vi "GetEnterExitLevelofPFLA.vi"(8 "error in (no error)":errorcluster, 10 "DataGroup":T1, 11 "PFLA Source":string) -> (0 "error out":errorcluster, 2 "ExitStartupPFLA%":dbl, 3 "EnterStartupPFLA%":dbl)   [LabVIEW 2017, in "McsaStartupAnalysis.lvlib"]
uses:
  <vilib>/addons/InsightCM/Devices/Shared/Mcsa/McsaStartupAnalysis/McsaStartupAnalysis.lvlib
  <vilib>/addons/InsightCM/MessageBus/Base/controls/R2_DataGroup.ctl
  <vilib>/addons/InsightCM/MessageBus/Base/controls/OperatingState.ctl
  <vilib>/addons/InsightCM/MessageBus/Base/controls/KeyValuePair.ctl
  <vilib>/addons/InsightCM/MessageBus/Base/controls/Trigger.ctl
  <vilib>/addons/InsightCM/MessageBus/Base/controls/Condition.ctl
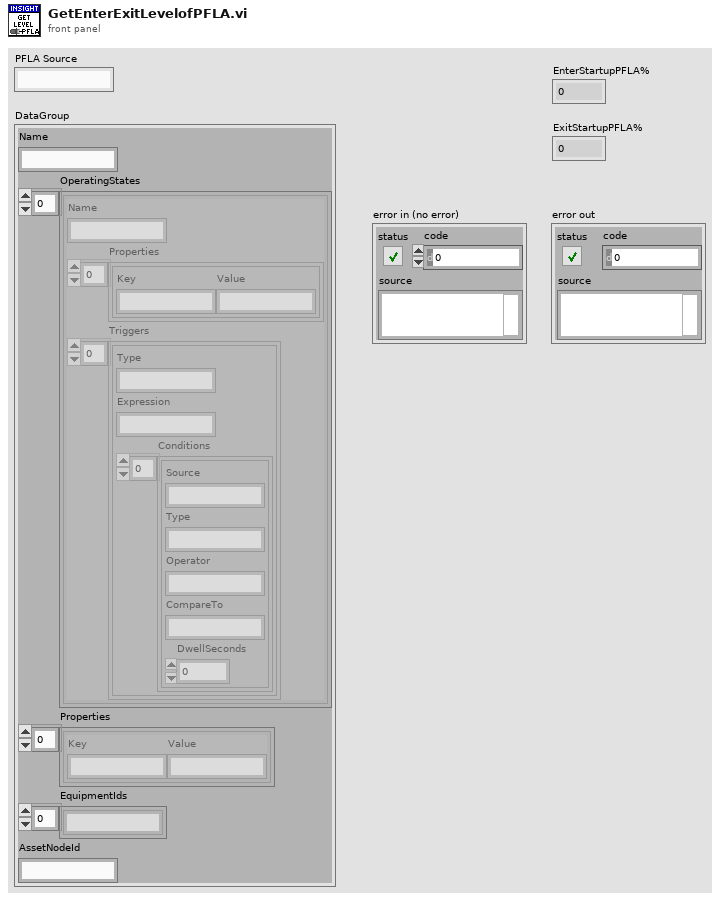
[diagram p1: front panel]
types:
  T1 = typedef "R2_DataGroup.ctl" = cluster{"Name":string, "OperatingStates":T2[], "Properties":T3[], "EquipmentIds":string[], "AssetNodeId":string}
  T2 = typedef "OperatingState.ctl" = cluster{"Name":string, "Properties":T3[], "Triggers":T4[]}
  T3 = typedef "KeyValuePair.ctl" = cluster{"Key":string, "Value":string}
  T4 = typedef "Trigger.ctl" = cluster{"Type":string, "Expression":string, "Conditions":T5[]}
  T5 = typedef "Condition.ctl" = cluster{"Source":string, "Type":string, "Operator":string, "CompareTo":string, "DwellSeconds":dbl}
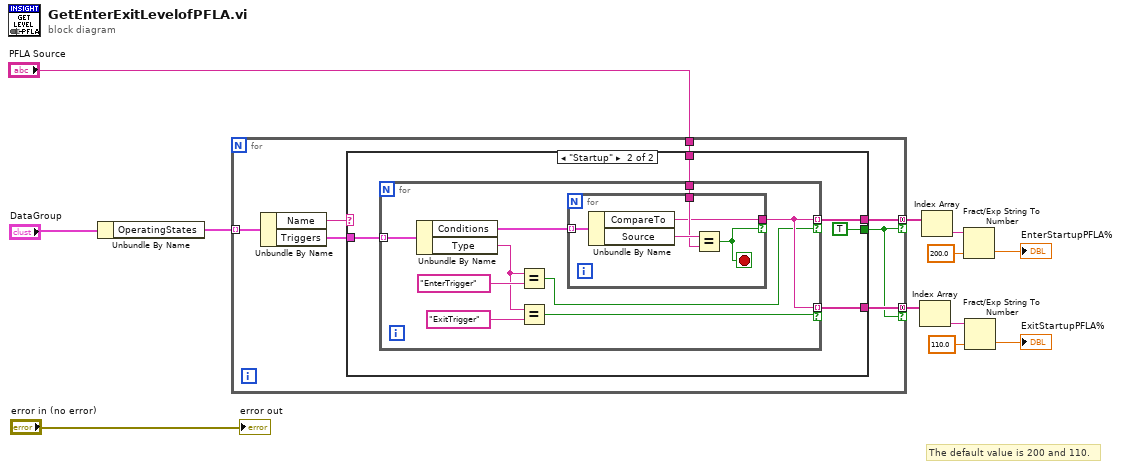
[diagram p0: block diagram]
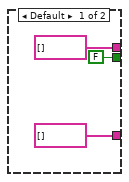
[diagram p2: hidden frame]
diagram:
  # "The default value is 200 and 110."
  n1 = Unbundle By Name("DataGroup") -> ("OperatingStates"=w3:T2[])
  n2 = for {
    tunnel: w3 -> [w19] mode=indexing
    tunnel: "PFLA Source" -> [w17]
    tunnel: [w15] -> w7 mode=concatenating if=w13
    tunnel: [w14] -> w8 mode=concatenating if=w13
    n3 = Unbundle By Name(w19) -> ("Name"=w16:string, "Triggers"=w18:T4[])
    n4 = case shown="\"Startup\"" w16 {
      tunnel: w18 -> [_ w27]
      tunnel: w17 -> [_ w26]
      tunnel: [string[] [] w25] -> w15
      tunnel: [string[] [] w24] -> w14
      tunnel: [FALSE ("x = y?") TRUE ("x = y?")] -> w13
      frame Default {
      }
      frame "Startup" {
        n5 = for {
          tunnel: w27 -> [w36] mode=indexing
          tunnel: w26 -> [w33]
          tunnel: [w30] -> w25 mode=indexing if=w29
          tunnel: [w30] -> w24 mode=indexing if=w28
          n6 = Unbundle By Name(w36) -> ("Conditions"=w34:T5[], "Type"=w31:string)
          n7 = Equal?(x=w31, y="EnterTrigger" ("Type")) -> (x = y?=w29:bool)
          n8 = Equal?(x=w31, y="ExitTrigger" ("Type")) -> (x = y?=w28:bool)
          n9 = for {
            tunnel: w34 -> [w41] mode=indexing
            tunnel: w33 -> [w39]
            tunnel: [w38] -> w30 if=w37
            stop <- w37 stop-if-true
            n10 = Unbundle By Name(w41) -> ("CompareTo"=w38:string, "Source"=w40:string)
            n11 = Equal?(x=w40, y=w39) -> (x = y?=w37:bool)
          }
        }
      }
    }
  }
  n12 = Index Array(array=w8) -> (element=w10:string)  [unwired: 1 in]
  n13 = Index Array(array=w7) -> (element=w9:string)  [unwired: 1 in]
  n14 = Fract/Exp String To Number(string=w9, default (0 dbl)=200.0 ("default (0 DBL)")) -> (number=→"EnterStartupPFLA%":dbl)  [unwired: 2 in, 1 out]
  n15 = Fract/Exp String To Number(string=w10, default (0 dbl)=110.0 ("default (0 DBL)")) -> (number=→"ExitStartupPFLA%":dbl)  [unwired: 2 in, 1 out]
  "error out" <- "error in (no error)"
